vi "Set Plot Properties.vi"(8 "error in (no error)":errorcluster, 10 "Plot Props":T1[](array[typedef]), 11 "Graph Refnum":refnum<vi>) -> (0 "error out":errorcluster)   [LabVIEW 2020]
uses:
  Plot Properties.ctl
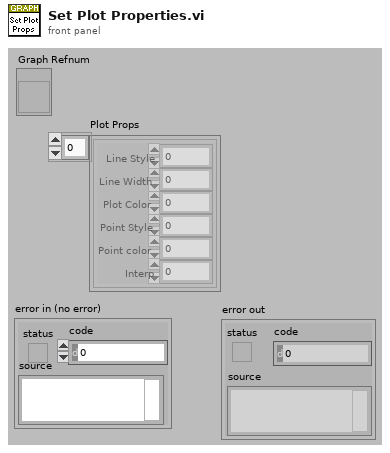
[diagram p1: front panel]
types:
  T1 = typedef "Plot Properties.ctl" = cluster{"Line Style":u8, "Line Width":u8, "Plot Color":u32, "Point Style":u8, "Point color":u32, "Interp":u8}
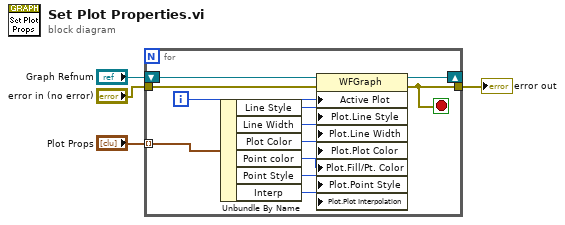
[diagram p0: block diagram]
diagram:
  n1 = for {
    tunnel: [w15] -> w4
    tunnel: "error in (no error)" -> [w13]
    tunnel: "Plot Props" -> [w12] mode=indexing
    shift-right: [w6] -> _
    shift-left: "Graph Refnum" -> [w14]
    i -> [w16]
    stop <- w15 stop-if-true
    n2 = Unbundle By Name(w12) -> ("Line Style"=w11:u8, "Line Width"=w10:u8, "Plot Color"=w9:u32, "Point color"=w8:u32, "Point Style"=w7:u8, "Interp"=w5:u8)
    n3 = property class="WFGraph"(reference=w14, error in=w13, "Active Plot"=w16, "Plot.Line Style"=w11, "Plot.Line Width"=w10, "Plot.Plot Color"=w9, "Plot.Fill/Pt. Color"=w8, "Plot.Point Style"=w7, "Plot.Plot Interpolation"=w5) -> (reference out=w6:refnum<vi>, error out=w15:errorcluster)
  }
  "error out" <- w4
